vi "ASK.vi"() -> ()   [LabVIEW 2016]
panel:
  out "sq":dynamicdata(graph) caption="Sine"
  out "Sine":dynamicdata(graph)
  out "ASK":dynamicdata(graph)
  in  "Sq freq":dbl(slide)=10.1 caption="Frequency" scale=0.0..100.0
  in  "sq amp":dbl(slide)=1.0 caption="Amplitude" scale=0.0..10.0
  in  "Frequency":dbl(slide)=10.1 scale=0.0..1000.0
  in  "Amplitude":dbl(slide)=1.0 scale=0.0..10.0
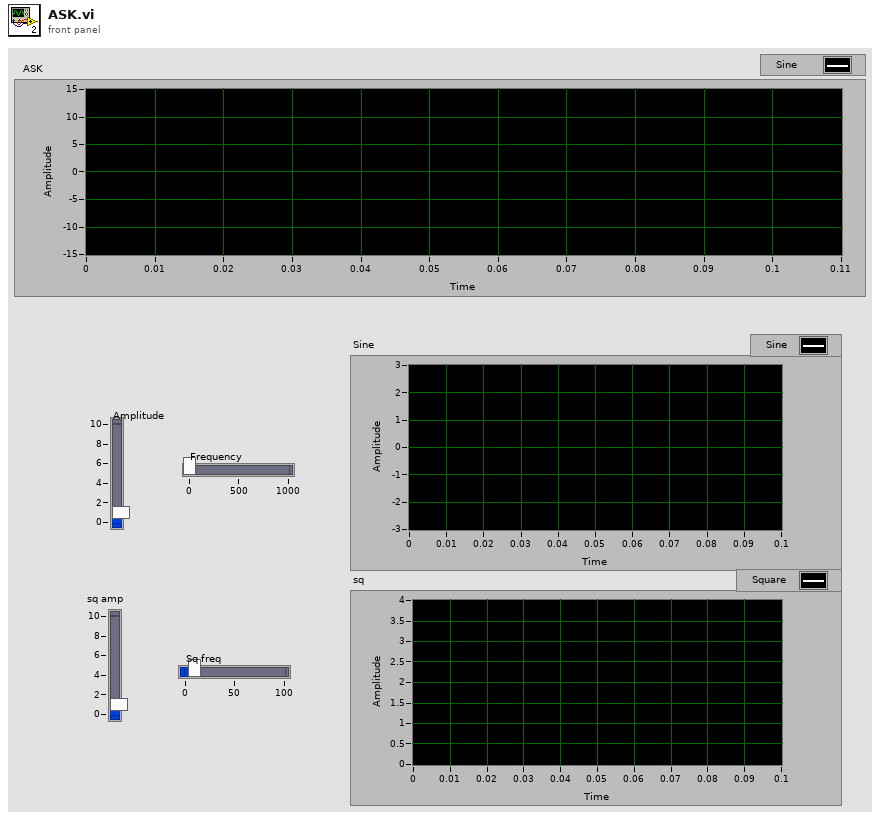
[diagram p1: front panel]
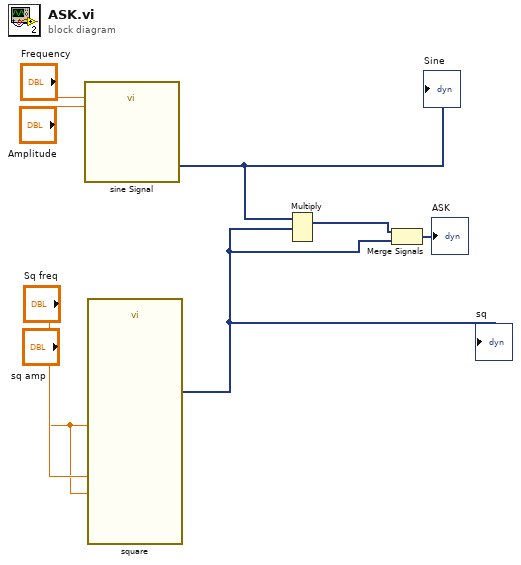
[diagram p0: block diagram]
diagram:
  n1 = call "sine Signal"("Frequency"="Frequency", "Amplitude"="Amplitude") -> ("Sine"=w5:dynamicdata)  [unwired: 12 in, 1 out]
  "Sine" <- w5
  n2 = call "square"("Offset"="sq amp", "Frequency"="Sq freq", "Amplitude"="sq amp") -> ("Square"=w3:dynamicdata)  [unwired: 11 in, 1 out]
  "sq" <- w3
  n3 = Multiply(1:w3, 2:w5) -> (0:w4:dynamicdata)  [unwired: 1 in, 1 out]
  n4 = Merge Signals(w4, w3) -> (→"ASK":dynamicdata)
